vi "write_log_metadata.vi"(8 "error in (no error)":errorcluster, 10 "data":variant, 11 "tt20_logger in":refnum<class "tt20_logger.lvclass">) -> (0 "error out":errorcluster, 3 "tt20_logger out":refnum<class "tt20_logger.lvclass">)   [LabVIEW 2015, in "tt20_logger.lvclass"]
uses:
  tt20_logger.lvclass
  tt20_logger.lvclass/tt20_logger.ctl
  <vilib>/UPVI/lvhdf5/attribute.llb/Simple H5Awrite (Variant).vi
  <vilib>/UPVI/lvhdf5/attribute.llb/LVH5A Operation.ctl
  <vilib>/UPVI/lvhdf5/attribute.llb/Simple H5Awrite.xnode
  <vilib>/UPVI/lvhdf5/library.llb/HDF5 Ref.ctl
  Picoquant/Hydraharp/hdf5_photon_record_logger/hdf5_photon_record_log.lvclass
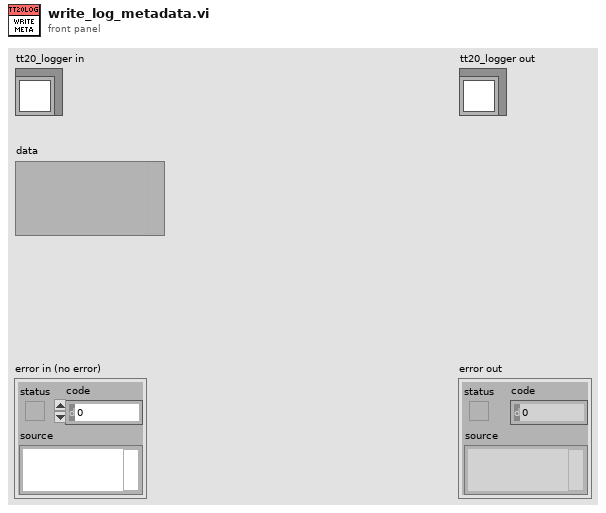
[diagram p1: front panel]
types:
  T1 = typedef "HDF5 Ref.ctl" = refnum<k1>
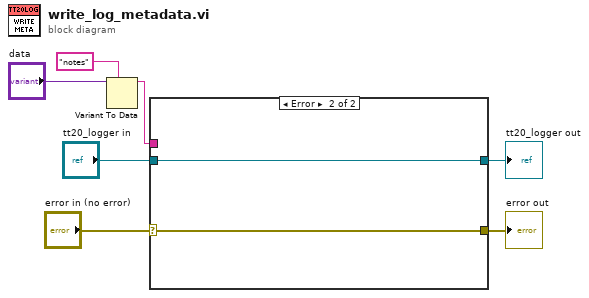
[diagram p0: block diagram]
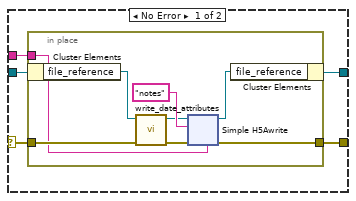
[diagram p2: hidden frame]
diagram:
  n1 = Variant To Data(type="notes" ("Name"), Variant="data") -> (data=w2:string)  [unwired: 1 in, 1 out]
  n2 = case shown="Error" "error in (no error)" {
    selector: "error in (no error)" -> [w11 w36]
    tunnel: "tt20_logger in" -> [w12 w37]
    tunnel: [w10 w36] -> w5
    tunnel: w2 -> [w9 _]
    tunnel: [w8 w37] -> w1
    frame No Error {
      n3 = in-place {
        in-place-border: w11 -> [w19]
        in-place-border: [w17] -> w10
        in-place-border: w9 -> [w15]
        n4 = in-place-cluster #1(w12) -> ("file_reference"=w20:T1)
        n5 = call "write_date_attributes.vi"("error in (no error)"=w19, "HDF5 Ref"=w20) -> ("error out"=w18:errorcluster, "HDF5 Ref out"=w14:T1)  [unwired: 8 in]
        n6 = xnode "Simple H5Awrite"("HDF5 Ref"=w14, "Name"="notes", "error in (no error)"=w18, "Value"=w15) -> ("HDF5 Ref out"=w13:T1, "error out"=w17:errorcluster)  [unwired: 1 in]
        n7 = in-place-cluster #1("file_reference"=w13) -> (w8:refnum<class "tt20_logger.lvclass">)
      }
    }
    frame Error {
    }
  }
  "tt20_logger out" <- w1
  "error out" <- w5
